vi "KepcoDCPwr Software Timed Ramp.vi"(0 "VISA resource name":refnum<visa-resource-name>, 1 "Disable @ End":bool, 2 "Repeat":bool, 3 "# of Cycles":i32, 4 "Model In":string, 5 "Start (Volts)":dbl format="%.2f", 6 "Boolean":bool=TRUE, 7 "End (Volts)":dbl format="%.2f", 9 "Voltage Increment":dbl format="%.2f", 11 "error in (no error)":errorcluster, 12 "Dwell (ms)":u32, 13 "Readback Voltage":bool, 14 "Readback Current":bool) -> (8 "End voltage":dbl, 15 "error out":errorcluster)   [LabVIEW 2013]
panel:
  in  "Stop 2":bool
  in  "Stop":bool
  out "Cycle Number":i32
  out "DC AMPERES":dbl format="%.3f"
  out "DC VOLTS":dbl format="%.3f"
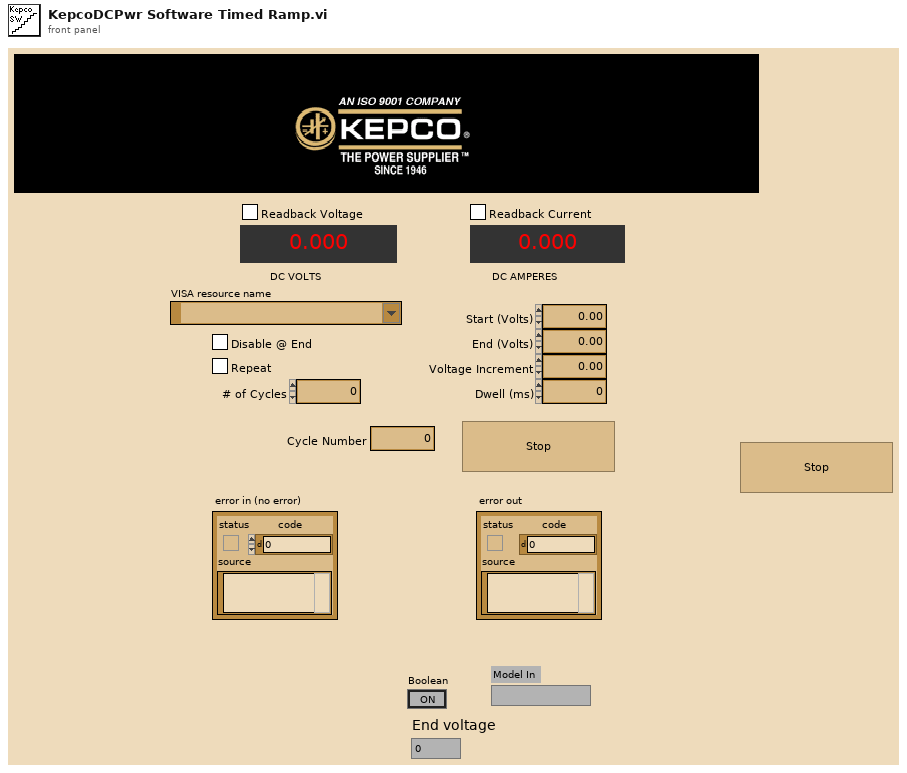
[diagram p1: front panel]
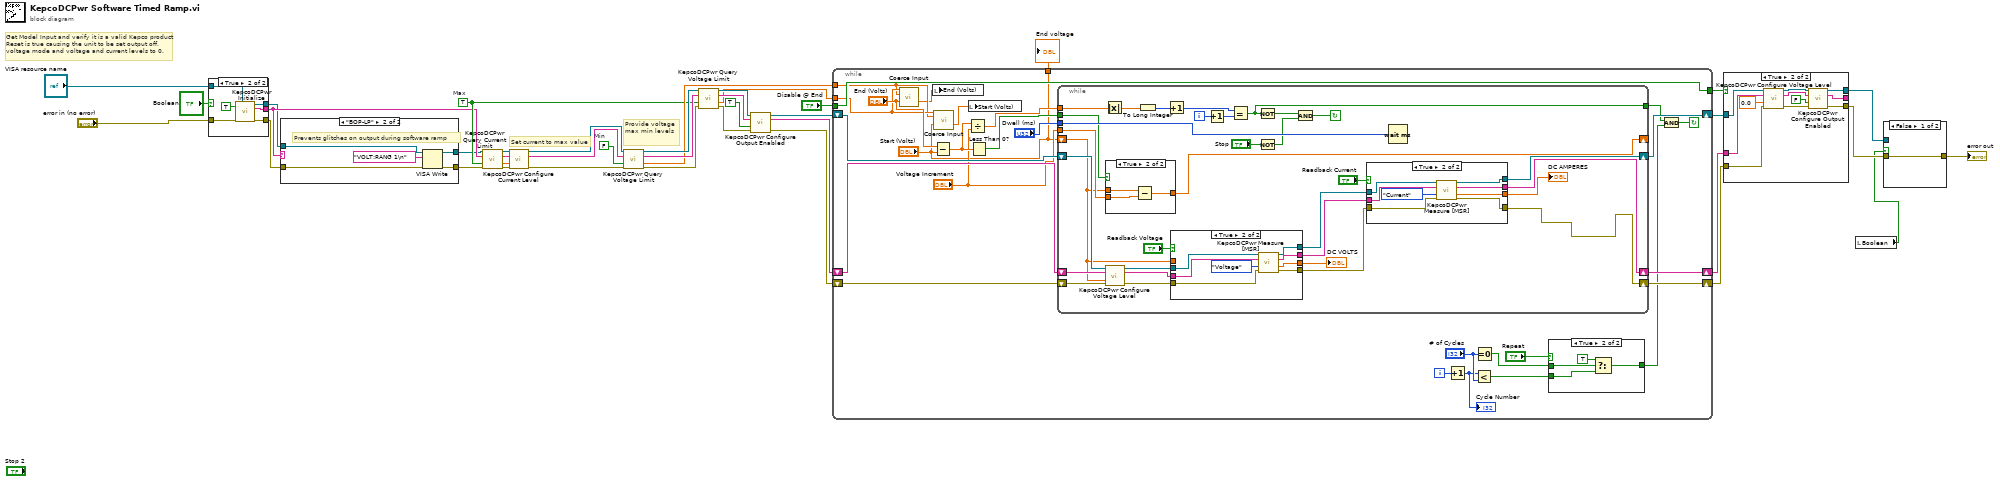
[diagram p0: block diagram]
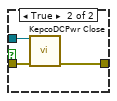
[diagram p2: hidden frame]
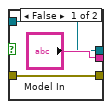
[diagram p3: hidden frame]
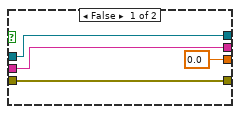
[diagram p5: hidden frame]
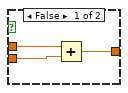
[diagram p7: hidden frame]
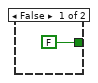
[diagram p8: hidden frame]
diagram:
  w17 = TRUE  # Max
  w23 = FALSE  # Min
  # "Provide voltage max min levels"
  # "Set current to max value"
  # "Get Model Input and verify it is a valid Kepco product Reset is true causing the unit to be set output off, voltage mode and voltage and current levels to 0."
  n1 = case shown="True" "Boolean" {
    tunnel: "error in (no error)" -> [w40 w47]
    tunnel: "VISA resource name" -> [w41 w46]
    tunnel: ["Model In" w45] -> w8
    tunnel: [w41 w44] -> w7
    tunnel: [w40 w43] -> w5
    frame False {
    }
    frame True {
      n2 = call "KepcoDCPwr Initialize.vi"("VISA Resource Name"=w46, "id query (True)"=TRUE, "error in (no error)"=w47) -> ("VISA Session Out"=w44:refnum<visa-resource-name>, "Model Out"=w45:string, "error out"=w43:errorcluster)  [unwired: 3 in, 7 out]
    }
  }
  n3 = case shown="\"BOP-LP\"" w8 {
    tunnel: w5 -> [w50 w55]
    tunnel: [w50 w52] -> w4
    tunnel: [w49 w53] -> w6
    tunnel: w7 -> [w49 w54]
    frame "", "STANDARD", Default {
    }
    frame "BOP-LP" {
      # "Prevents glitches on output during software ramp"
      n4 = VISA Write(VISA resource name=w54, write buffer="VOLT:RANG 1\n", error in (no error)=w55) -> (VISA resource name out=w53:refnum<visa-resource-name>, error out=w52:errorcluster)  [unwired: 1 out]
    }
  }
  n5 = call "KepcoDCPwr Query Current Limit.vi"("VISA Session"=w6, "Model In"=w8, "Level"=w17, "error in (no error)"=w4) -> ("VISA Session Out"=w14:refnum<visa-resource-name>, "Model Out"=w11:string, "current limit"=w10:dbl, "error out"=w16:errorcluster)  [unwired: 1 in, 7 out]
  n6 = call "KepcoDCPwr Configure Current Level.vi"("VISA Session"=w14, "Model In"=w11, "level (0.0 volts)"=w10, "error in (no error)"=w16) -> ("VISA Session Out"=w13:refnum<visa-resource-name>, "Model Out"=w12:string, "error out"=w15:errorcluster)  [unwired: 1 in, 8 out]
  n7 = call "KepcoDCPwr Query Voltage Limit.vi"("VISA Session"=w13, "Model In"=w12, "Max Level (T),MIN LEVEL(F)"=w23, "error in (no error)"=w15) -> ("VISA Session Out"=w24:refnum<visa-resource-name>, "Model Out"=w25:string, "voltage level"=w18:dbl, "error out"=w26:errorcluster)  [unwired: 1 in, 7 out]
  n8 = call "KepcoDCPwr Query Voltage Limit.vi"("VISA Session"=w24, "Model In"=w25, "Max Level (T),MIN LEVEL(F)"=w17, "error in (no error)"=w26) -> ("VISA Session Out"=w22:refnum<visa-resource-name>, "Model Out"=w21:string, "voltage level"=w19:dbl, "error out"=w20:errorcluster)  [unwired: 1 in, 7 out]
  n9 = call "KepcoDCPwr Configure Output Enabled.vi"("VISA Session"=w22, "Model In"=w21, "Input enabled (True)"=TRUE, "error in (no error)"=w20) -> ("VISA Session Out"=w29:refnum<visa-resource-name>, "Model Out"=w31:string, "error out"=w30:errorcluster)  [unwired: 9 out]
  n10 = while {
    tunnel: w18 -> [w64]
    tunnel: w19 -> [w65]
    tunnel: [w78] -> w33
    tunnel: "Disable @ End" -> [w78]
    shift-left: w31 -> [w76]
    shift-right: [w80] -> w37
    shift-left: w30 -> [w75]
    shift-right: [w79] -> w36
    shift-left: w29 -> [w77]
    shift-right: [w81] -> w38
    tunnel: ["Start (Volts)"] -> w1
    i -> [w60]
    stop <- w69 continue-if-true
    n11 = call "Coerce Input.vi"("Max"=w65, "Min"=w64, "Input"="End (Volts)") -> ("Output"=w63:dbl)  [unwired: 12 out]
    n12 = local write "End (Volts)"(w63) -> ()
    n13 = Subtract(x="End (Volts)", y="Start (Volts)") -> (x-y=w73:dbl)
    n14 = call "Coerce Input.vi"("Max"=w65, "Min"=w64, "Input"="Start (Volts)") -> ("Output"=w67:dbl)  [unwired: 12 out]
    n15 = local write "Start (Volts)"(w67) -> ()
    n16 = Divide(x=w73, y="Voltage Increment") -> (x/y=w71:dbl)
    n17 = Less Than 0?(x=w73) -> (x < 0?=w72:bool)
    n18 = while {
      tunnel: [w83] -> w68
      tunnel: w71 -> [w104]
      tunnel: w72 -> [w107]
      tunnel: "Voltage Increment" -> [w109]
      shift-left: "Start (Volts)" -> [w103]
      shift-right: [w108] -> _
      tunnel: "Dwell (ms)" -> [w110]
      shift-left: w76 -> [w111]
      shift-right: [w95] -> w80
      shift-left: w77 -> [w112]
      shift-right: [w94] -> w81
      shift-left: w75 -> [w114]
      shift-right: [w113] -> w79
      i -> [w91]
      stop <- w88 continue-if-true
      n19 = Absolute Value(x=w104) -> (abs(x)=w105:dbl)
      n20 = case shown="True" w107 {
        tunnel: w103 -> [w140 w144]
        tunnel: w109 -> [w139 w143]
        tunnel: [w141 w142] -> w108
        frame False {
          n21 = Add(x=w140, y=w139) -> (x+y=w141:dbl)
        }
        frame True {
          n22 = Subtract(x=w144, y=w143) -> (x-y=w142:dbl)
        }
      }
      n23 = call "KepcoDCPwr Configure Voltage Level.vi"("VISA Session"=w112, "Model In"=w111, "level (0.0 volts)"=w103, "error in (no error)"=w114) -> ("VISA Session Out"=w101:refnum<visa-resource-name>, "Model Out"=w100:string, "error out"=w99:errorcluster)  [unwired: 1 in, 8 out]
      n24 = To Long Integer(number=w105) -> (32bit integer=w106:i32)
      n25 = Increment(x=w106) -> (x+1=w92:i32)
      n26 = case shown="True" "Readback Voltage" {
        tunnel: w103 -> [w130 _]
        tunnel: [w130 w132] -> w102
        tunnel: w101 -> [w129 w134]
        tunnel: w100 -> [w128 w136]
        tunnel: w99 -> [w127 w138]
        tunnel: [w129 w133] -> w98
        tunnel: [w128 w135] -> w97
        tunnel: [w127 w137] -> w96
        frame False {
        }
        frame True {
          n27 = call "KepcoDCPwr Measure [MSR].vi"("VISA Session"=w134, "Model In"=w136, "measurement type (voltage)"=enum16{"Voltage", "Current"}."Voltage", "error in (no error)"=w138) -> ("VISA Session Out"=w133:refnum<visa-resource-name>, "Model Out"=w135:string, "measurement"=w132:dbl, "error out"=w137:errorcluster)  [unwired: 4 in, 4 out]
        }
      }
      "DC VOLTS" <- w102
      n28 = Increment(x=w91) -> (x+1=w90:i32)
      n29 = Equal?(x=w92, y=w90) -> (x = y?=w83:bool)
      n30 = Not(x=w83) -> (.not. x?=w89:bool)
      n31 = Not(x="Stop") -> (.not. x?=w87:bool)
      n32 = And(x=w89, y=w87) -> (x .and. y?=w88:bool)
      n33 = case shown="True" "Readback Current" {
        tunnel: [0.0 ("measurement") w120] -> w93
        tunnel: w98 -> [w118 w122]
        tunnel: w97 -> [w117 w124]
        tunnel: w96 -> [w116 w126]
        tunnel: [w118 w121] -> w94
        tunnel: [w117 w123] -> w95
        tunnel: [w116 w125] -> w113
        frame False {
        }
        frame True {
          n34 = call "KepcoDCPwr Measure [MSR].vi"("VISA Session"=w122, "Model In"=w124, "measurement type (voltage)"=enum16{"Voltage", "Current"}."Current", "error in (no error)"=w126) -> ("VISA Session Out"=w121:refnum<visa-resource-name>, "Model Out"=w123:string, "measurement"=w120:dbl, "error out"=w125:errorcluster)  [unwired: 4 in, 4 out]
        }
      }
      "DC AMPERES" <- w93
      n35 = Wait (ms)(milliseconds to wait=w110) -> ()  [unwired: 1 out]
    }
    n36 = Increment(x=w60) -> (x+1=w58:i32)
    "Cycle Number" <- w58
    n37 = Less?(x=w58, y="# of Cycles") -> (x < y?=w82:bool)
    n38 = Equal To 0?(x="# of Cycles") -> (x = 0?=w62:bool)
    n39 = case shown="True" "Repeat" {
      tunnel: [FALSE w148] -> w70
      tunnel: w82 -> [_ w146]
      tunnel: w62 -> [_ w149]
      frame False {
      }
      frame True {
        n40 = Select(t=TRUE ("f"), s=w149, f=w146) -> (s? t:f=w148:bool)
      }
    }
    n41 = And(x=w68, y=w70) -> (x .and. y?=w69:bool)
  }
  "End voltage" <- w1
  n42 = case shown="True" w33 {
    tunnel: w38 -> [w152 w163]
    tunnel: w37 -> [w151 w162]
    tunnel: w36 -> [w150 w161]
    tunnel: [w150 w156] -> w34
    tunnel: [w152 w155] -> w35
    tunnel: [w151 w154] -> _
    frame False {
    }
    frame True {
      n43 = call "KepcoDCPwr Configure Voltage Level.vi"("VISA Session"=w163, "Model In"=w162, "level (0.0 volts)"=0.0, "error in (no error)"=w161) -> ("VISA Session Out"=w159:refnum<visa-resource-name>, "Model Out"=w158:string, "error out"=w157:errorcluster)  [unwired: 1 in, 8 out]
      n44 = call "KepcoDCPwr Configure Output Enabled.vi"("VISA Session"=w159, "Model In"=w158, "Input enabled (True)"=FALSE ("output enabled (True)"), "error in (no error)"=w157) -> ("VISA Session Out"=w155:refnum<visa-resource-name>, "Model Out"=w154:string, "error out"=w156:errorcluster)  [unwired: 9 out]
    }
  }
  n45 = local read "Boolean"() -> (w2:bool)
  n46 = case shown="False" w2 {
    tunnel: w35 -> [_ w167]
    tunnel: w34 -> [w164 w166]
    tunnel: [w164 w165] -> w28
    frame False {
    }
    frame True {
      n47 = call "KepcoDCPwr Close.vi"("VISA Session"=w167, "error in (no error)"=w166) -> ("error out"=w165:errorcluster)  [unwired: 13 out]
    }
  }
  "error out" <- w28
